vi "Struve Function.vi"(2 "v":dbl format="%.2f", 3 "x":dbl format="%.2f") -> (1 "Hv(x)":dbl format="%.2f")   [LabVIEW 2014, in "NI_Gmath.lvlib"]
doc: "Computes the Struve function."
uses:
  NI_Gmath.lvlib
  lvanlys.dll
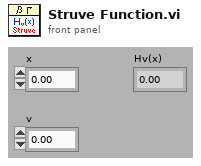
[diagram p1: front panel]
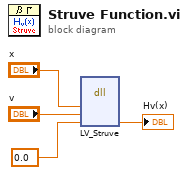
[diagram p0: block diagram]
diagram:
  n1 = dll-call lib="C:/Program Files (x86)/National Instruments/LabVIEW 2014/resource/lvanlys.*" fn="LV_Struve"("x"="x", "v"="v", "Struve(x, v)"=0.0 ("cylinder")) -> ("Struve(x, v)"=→"Hv(x)":dbl)  [unwired: 6 in, 2 out]
